vi "LDT Telescope Config GUI.vi"(11 "LDT Telescope Settings":T1={"host"="localhost", "port"="61616"}) -> (2 "cancelled":bool, 3 "LDT Telescope Settings out":T1={"host"="localhost", "port"="61616"})   [LabVIEW 2022 SP3, in "LDT Telescope.lvclass"]
uses:
  LDT Telescope.lvclass
  typedef cluster LDT Telescope Settings.ctl
panel:
  in  "Standard Settings":enum16{"Simulation", "Lowell Telescope"}(ring)
  in  "Cancel Button":bool
  in  "Save":bool
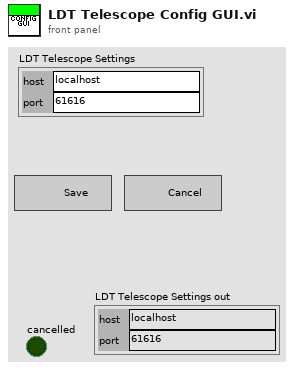
[diagram p1: front panel]
types:
  T1 = typedef "LDT Telescope.lvclass/typedef cluster LDT Telescope Settings.ctl" = cluster{"host":string, "port":string}
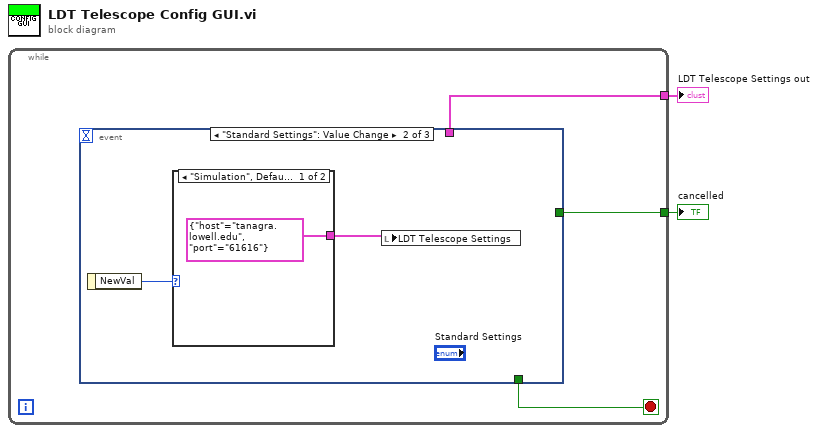
[diagram p0: block diagram]
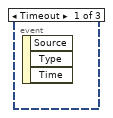
[diagram p2: hidden frame]
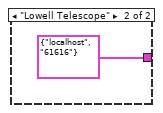
[diagram p3: hidden frame]
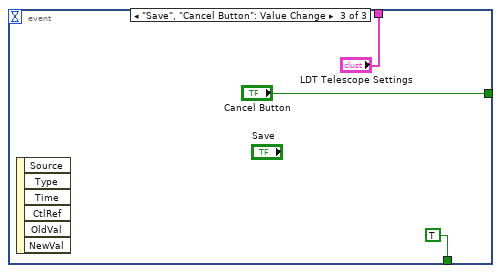
[diagram p4: hidden frame]
diagram:
  n1 = while {
    tunnel: [w4] -> w2
    tunnel: [w3] -> w1
    stop <- w5 stop-if-true
    n2 = event shown="[1] \"Standard Settings\": Value Change" {
      selector: _ -> [_ _ _]
      dyn-events: _ -> [_ _ _]
      timeout: _ -> [_ _ _]
      tunnel: [_ _ TRUE] -> w5
      tunnel: [_ _ "Cancel Button"] -> w4
      tunnel: [_ _ "LDT Telescope Settings"] -> w3
      event Timeout {
        n3 = event-data() -> ()  [unwired: 1 in, 3 out]
      }
      event "Standard Settings": Value Change {
        n4 = event-data() -> ("NewVal"=w7:enum16{"Simulation", "Lowell Telescope"})  [unwired: 1 in]
        n5 = case shown="\"Simulation\", Default" w7 {
          tunnel: [T1 {"host"="tanagra.lowell.edu", "port"="61616"} ("LDT Telescope Settings") T1 {"host"="localhost", "port"="61616"} ("LDT Telescope Settings")] -> w6
          frame "Simulation", Default {
          }
          frame "Lowell Telescope" {
          }
        }
        n6 = local write "LDT Telescope Settings"(w6) -> ()
      }
      event "Save", "Cancel Button": Value Change {
        n7 = event-data() -> ()  [unwired: 1 in, 6 out]
      }
    }
  }
  "cancelled" <- w2
  "LDT Telescope Settings out" <- w1
